vi "init wave.vi"(9 "chanelcouter":i32, 10 "t0":timestamp, 11 "dt":dbl) -> (2 "initialized array":waveform(dbl)[](array[waveform]))   [LabVIEW 2009]
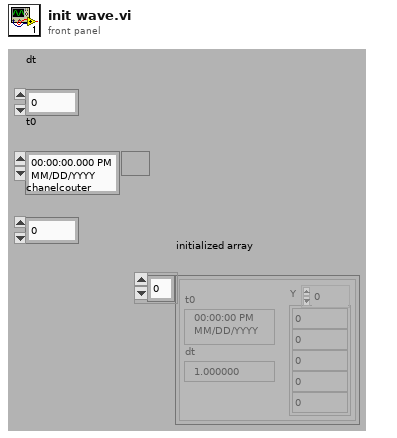
[diagram p1: front panel]
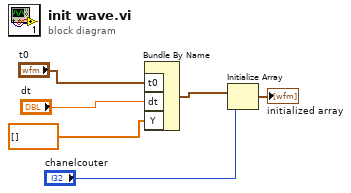
[diagram p0: block diagram]
diagram:
  n1 = Bundle By Name("t0"="t0", "dt"="dt", "Y"=dbl[] []) -> (w6:waveform(dbl))  [unwired: 1 out]
  n2 = Initialize Array(w6, "chanelcouter") -> (→"initialized array":waveform(dbl)[])
